vi "AnalogOUT_Normieren.vi"(7 "Analogwert":sgl, 8 "Obergrenze":sgl, 9 "Untergrenze":sgl, 10 "Max Analogwert":sgl, 11 "Min Analogwert":sgl) -> (2 "Normierter Wert":sgl)   [LabVIEW 2020, in "Verwaltung - cRIO.lvlib"]
uses:
  Verwaltung - cRIO.lvlib
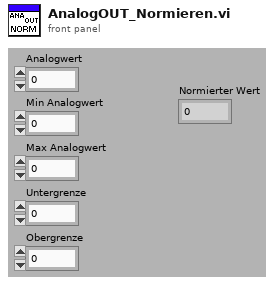
[diagram p1: front panel]
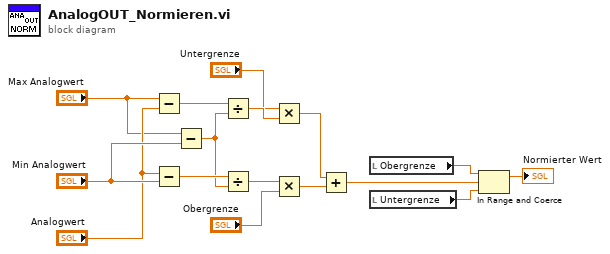
[diagram p0: block diagram]
diagram:
  n1 = Subtract(x="Max Analogwert", y="Analogwert") -> (x-y=w16:sgl)
  n2 = Subtract(x="Analogwert", y="Min Analogwert") -> (x-y=w15:sgl)
  n3 = Subtract(x="Max Analogwert", y="Min Analogwert") -> (x-y=w14:sgl)
  n4 = Divide(x=w16, y=w14) -> (x/y=w13:sgl)
  n5 = Divide(x=w15, y=w14) -> (x/y=w12:sgl)
  n6 = Multiply(x="Untergrenze", y=w13) -> (x*y=w8:sgl)
  n7 = Multiply(x=w12, y="Obergrenze") -> (x*y=w9:sgl)
  n8 = Add(x=w8, y=w9) -> (x+y=w4:sgl)
  n9 = local read "Obergrenze"() -> (w3:sgl)
  n10 = local read "Untergrenze"() -> (w2:sgl)
  n11 = In Range and Coerce(upper limit=w3, x=w4, lower limit=w2) -> (coerced(x)=→"Normierter Wert":sgl)  [unwired: 1 out]
